vi "Compare_values_Modify_Cost_f()-2.vi"(4 "error IN":errorcluster, 5 "[IN] Cost function":i8[](array[numeric]), 6 "[IN] Additions to cost":i8[](array[numeric]), 7 "[IN] Array of displa\ncement differences":dbl[](array[numeric]), 8 "[IN] Statuses of points":i16[](array[numeric]), 9 "[IN] Areas \ndifferences":dbl[](array[numeric]), 10 "[IN] Reverse or not":bool[](array[boolean]), 11 "[IN] Angles betwe\nen displacements":dbl[](array[numeric])) -> (0 "error OUT":errorcluster, 3 "[OUT] Cost function":i8[](array[numeric]))   [LabVIEW 2013]
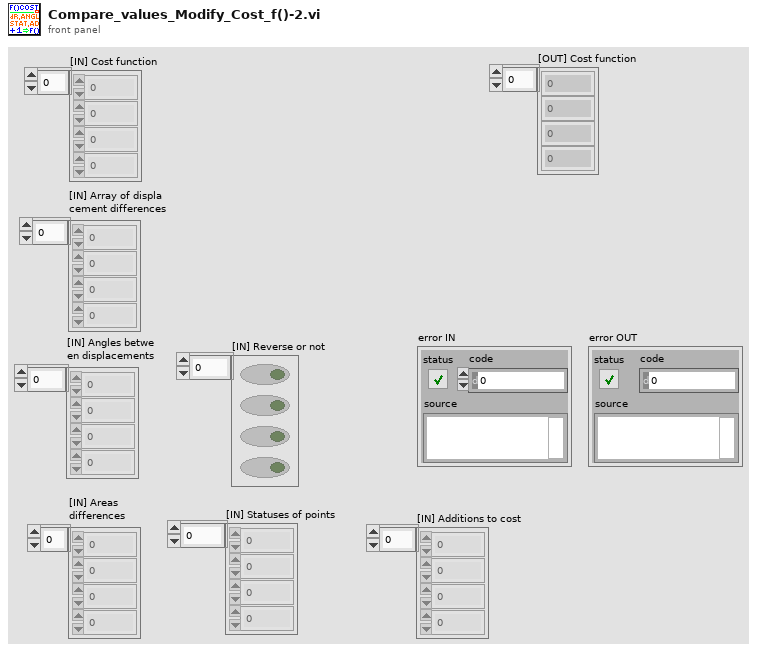
[diagram p1: front panel]
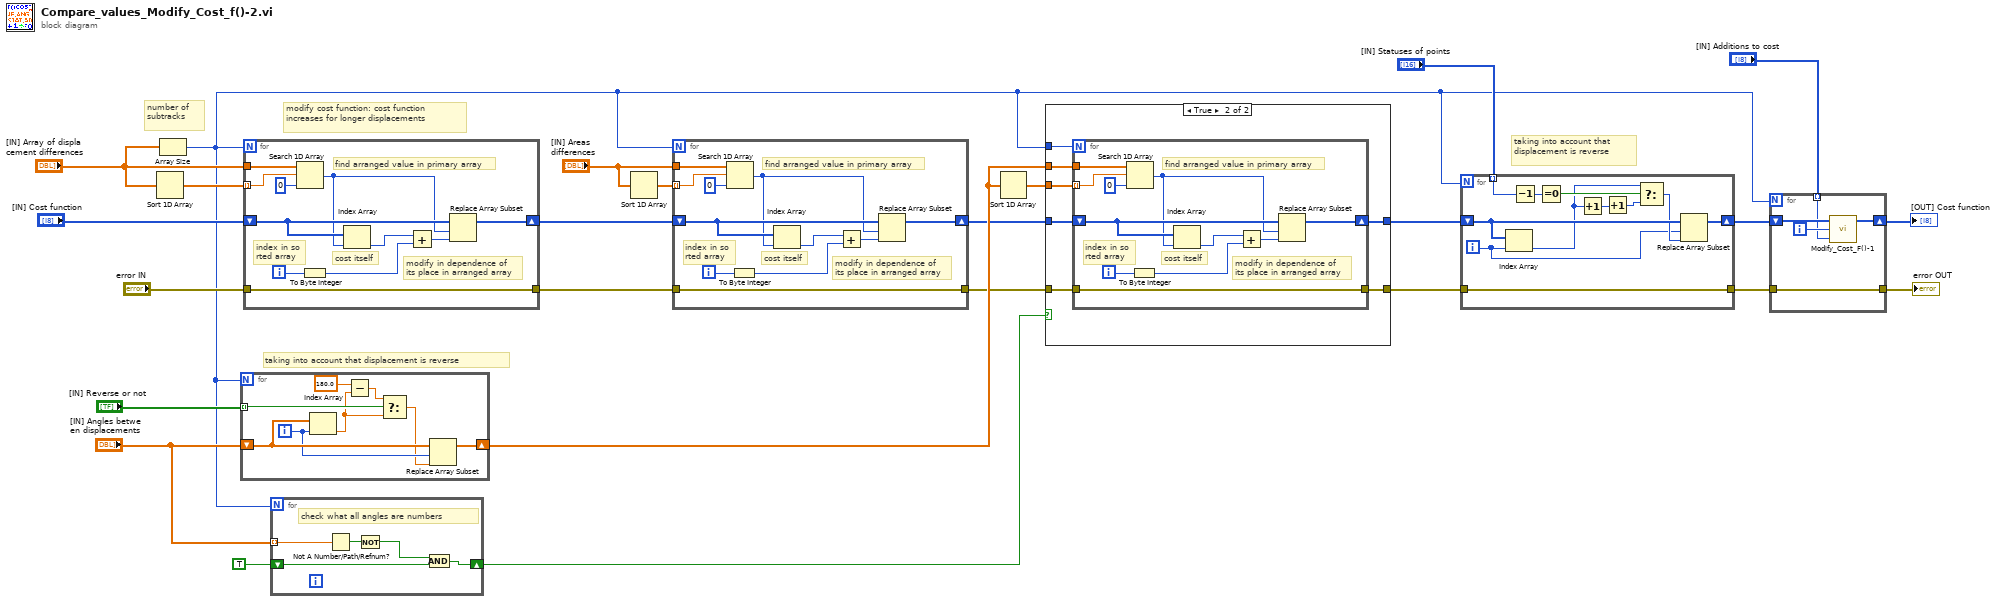
[diagram p0: block diagram]
diagram:
  # "taking into account that \ndisplacement is reverse"
  # "taking into account that displacement is reverse"
  # "modify cost function: cost function \nincreases for longer displacements"
  # "number of \nsubtracks"
  n1 = Sort 1D Array(array="[IN] Array of displa\ncement differences") -> (sorted array=w25:dbl[])
  n2 = Array Size(array="[IN] Array of displa\ncement differences") -> (size(s)=w2:i32)
  n3 = for {
    N: w2 -> [_]
    shift-right: [w26] -> w17
    shift-left: "[IN] Angles betwe\nen displacements" -> [w32]
    tunnel: "[IN] Reverse or not" -> [w33] mode=indexing
    i -> [w28]
    n4 = Index Array(array=w32, index=w28) -> (element=w30:dbl)
    n5 = Subtract(x=180.0, y=w30) -> (x-y=w29:dbl)
    n6 = Select(t=w29, s=w33, f=w30) -> (s? t:f=w27:dbl)
    n7 = Replace Array Subset(array=w32, new element=w27, index=w28) -> (w26:dbl[])
  }
  n8 = for {
    N: w2 -> [_]
    tunnel: w25 -> [w42] mode=indexing
    tunnel: "[IN] Array of displa\ncement differences" -> [w44]
    shift-right: [w35] -> w22
    shift-left: "[IN] Cost function" -> [w41]
    tunnel: "error IN" -> [w34]
    tunnel: [w34] -> w9
    i -> [w37]
    # "modify in dependence of \nits place in arranged array"
    # "find arranged value in primary array"
    # "index in so\nrted array"
    # "cost itself"
    n9 = Search 1D Array(1D array=w44, element=w42, start index (0)=0) -> (index of element=w40:i32)
    n10 = To Byte Integer(number=w37) -> (8bit integer=w36:i8)
    n11 = Index Array(array=w41, index=w40) -> (element=w39:i8)
    n12 = Add(x=w39, y=w36) -> (x+y=w38:i8)
    n13 = Replace Array Subset(array=w41, new element=w38, index=w40) -> (w35:i8[])
  }
  n14 = for {
    N: w2 -> [_]
    tunnel: "[IN] Angles betwe\nen displacements" -> [w48] mode=indexing
    shift-right: [w45] -> w1
    shift-left: TRUE -> [w49]
    # "check what all angles are numbers"
    n15 = Not A Number/Path/Refnum?(number/path/refnum=w48) -> (NaN/Path/Refnum?=w47:bool)
    n16 = Not(x=w47) -> (.not. x?=w46:bool)
    n17 = And(x=w46, y=w49) -> (x .and. y?=w45:bool)
  }
  n18 = Sort 1D Array(array="[IN] Areas \ndifferences") -> (sorted array=w20:dbl[])
  n19 = for {
    N: w2 -> [_]
    tunnel: w20 -> [w58] mode=indexing
    tunnel: "[IN] Areas \ndifferences" -> [w60]
    shift-right: [w51] -> w16
    shift-left: w22 -> [w57]
    tunnel: w9 -> [w50]
    tunnel: [w50] -> w8
    i -> [w53]
    # "modify in dependence of \nits place in arranged array"
    # "find arranged value in primary array"
    # "index in so\nrted array"
    # "cost itself"
    n20 = Search 1D Array(1D array=w60, element=w58, start index (0)=0) -> (index of element=w56:i32)
    n21 = To Byte Integer(number=w53) -> (8bit integer=w52:i8)
    n22 = Index Array(array=w57, index=w56) -> (element=w55:i8)
    n23 = Add(x=w55, y=w52) -> (x+y=w54:i8)
    n24 = Replace Array Subset(array=w57, new element=w54, index=w56) -> (w51:i8[])
  }
  n25 = Sort 1D Array(array=w17) -> (sorted array=w18:dbl[])
  n26 = case shown="True" w1 {
    tunnel: w18 -> [_ w69]
    tunnel: w17 -> [_ w68]
    tunnel: w16 -> [w62 w67]
    tunnel: [w62 w66] -> w15
    tunnel: w2 -> [_ w65]
    tunnel: w8 -> [w61 w64]
    tunnel: [w61 w63] -> w7
    frame False {
    }
    frame True {
      n27 = for {
        N: w65 -> [_]
        tunnel: w69 -> [w78] mode=indexing
        tunnel: w68 -> [w80]
        shift-right: [w71] -> w66
        shift-left: w67 -> [w77]
        tunnel: w64 -> [w70]
        tunnel: [w70] -> w63
        i -> [w73]
        # "modify in dependence of \nits place in arranged array"
        # "find arranged value in primary array"
        # "index in so\nrted array"
        # "cost itself"
        n28 = Search 1D Array(1D array=w80, element=w78, start index (0)=0) -> (index of element=w76:i32)
        n29 = To Byte Integer(number=w73) -> (8bit integer=w72:i8)
        n30 = Index Array(array=w77, index=w76) -> (element=w75:i8)
        n31 = Add(x=w75, y=w72) -> (x+y=w74:i8)
        n32 = Replace Array Subset(array=w77, new element=w74, index=w76) -> (w71:i8[])
      }
    }
  }
  n33 = for {
    N: w2 -> [_]
    shift-right: [w82] -> w13
    shift-left: w15 -> [w91]
    tunnel: "[IN] Statuses of points" -> [w90] mode=indexing
    tunnel: w7 -> [w81]
    tunnel: [w81] -> w6
    i -> [w83]
    n34 = Index Array(array=w91, index=w83) -> (element=w87:i8)
    n35 = Decrement(x=w90) -> (x-1=w89:i16)
    n36 = Equal To 0?(x=w89) -> (x = 0?=w88:bool)
    n37 = Increment(x=w87) -> (x+1=w86:i8)
    n38 = Increment(x=w86) -> (x+1=w85:i8)
    n39 = Select(t=w87, s=w88, f=w85) -> (s? t:f=w84:i8)
    n40 = Replace Array Subset(array=w91, new element=w84, index=w83) -> (w82:i8[])
  }
  n41 = for {
    N: w2 -> [_]
    shift-right: [w93] -> w11
    shift-left: w13 -> [w96]
    tunnel: "[IN] Additions to cost" -> [w94] mode=indexing
    tunnel: w6 -> [w92]
    tunnel: [w92] -> w5
    i -> [w95]
    n42 = call "Modify_Cost_F()-1.vi"("[IN] Additions to cost"=w94, "[IN] Current Index"=w95, "[IN] Cost function"=w96) -> ("[OUT] Cost function"=w93:i8[])  [unwired: 2 in]
  }
  "[OUT] Cost function" <- w11
  "error OUT" <- w5
